vi "Update String Value.vi"(10 "Tree Tag":string, 11 "UI Data In":refnum<class "Settings UI.lvclass">) -> (2 "New Tree Value":string, 3 "UI Data Out":refnum<class "Settings UI.lvclass">)   [LabVIEW 2020, in "Output Sequencer.lvlib" / "Settings UI.lvclass"]
uses:
  Settings UI.lvclass
  Settings UI.lvclass/Settings UI.ctl
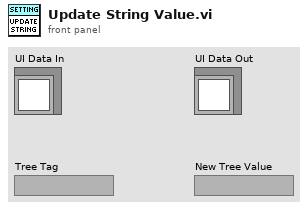
[diagram p1: front panel]
types:
  T1 = typedef "Output Sequencer.lvlib/Settings UI.lvclass/Tree Index Enum.ctl" = enum16{"General Settings", "Num Steps", "Num Analog", "Num Digital", "Show Confirmation", "Interp Priority", "Adv Timing", "Enable Conditions", "Seq Execution", "Reset Test Start", "Only When Test", "Delay After Test", "Start condition", "Re-triggering", "Stop condition", "Stop After Cycles", "Stop Values", "Default Values", "Default Analog", "Default Digital", "Steps", "Step #", "Description", "Precondition", "Duration", "Mode", "Delay Between Vals", "Analog Values", "Digital Values", "Postcondition", "On True", "On False"}
  T2 = typedef "Output Sequencer.lvlib/Settings UI.lvclass/Step Settings.ctl" = cluster{"Description":string, "Precondition":string, "Duration":dbl, "Mode":string, "Delay Between Values":dbl, "Analog Values":string[], "Digital Values":string[], "Postcondition":string, "On True":string, "On False":string}
  T3 = map{i32, cluster{"Step Number":i32, "Description":string}}
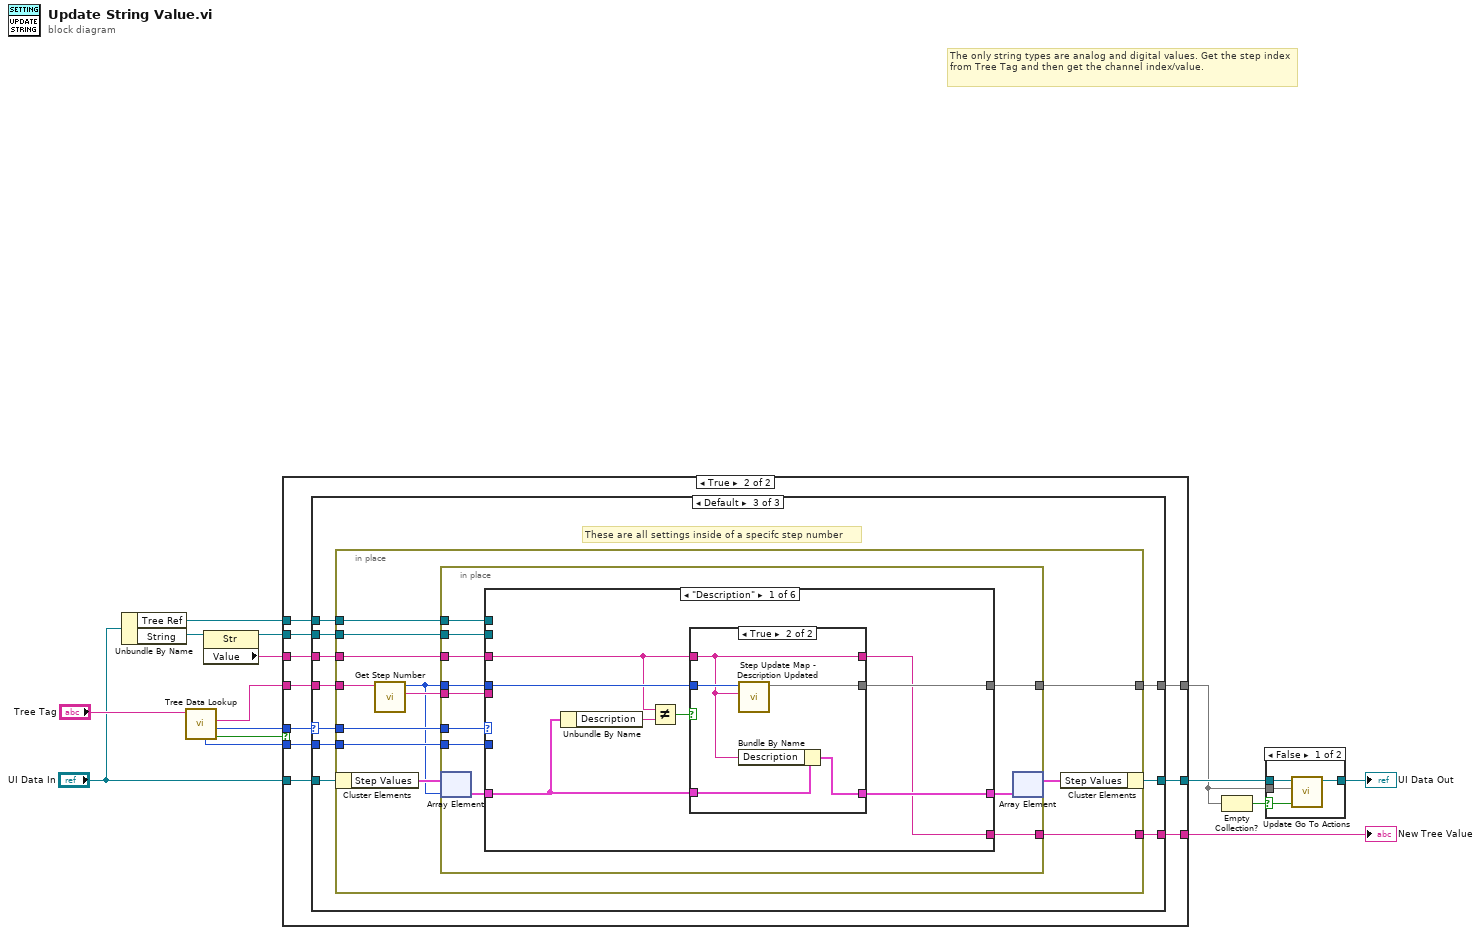
[diagram p0: block diagram]
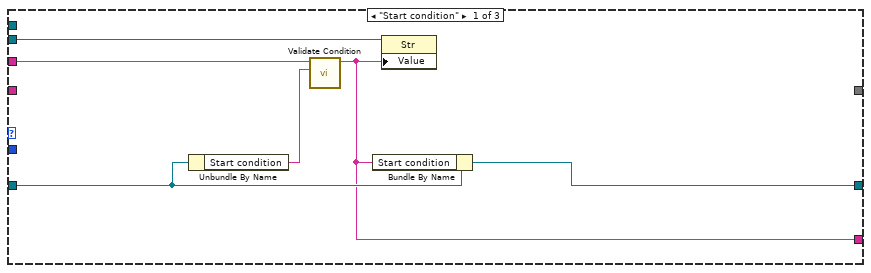
[diagram p4: hidden frame]
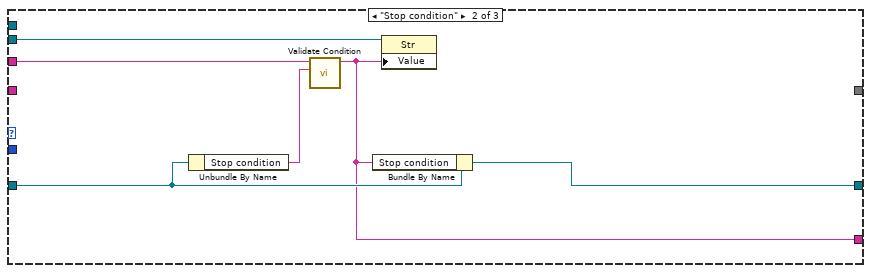
[diagram p5: hidden frame]
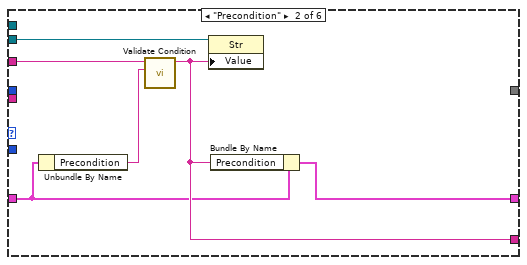
[diagram p7: hidden frame]
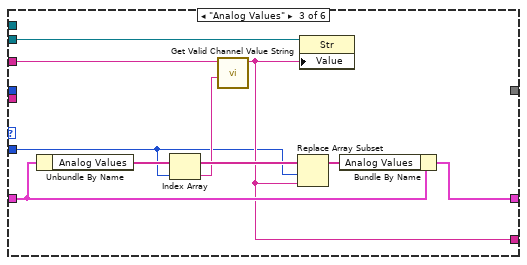
[diagram p8: hidden frame]
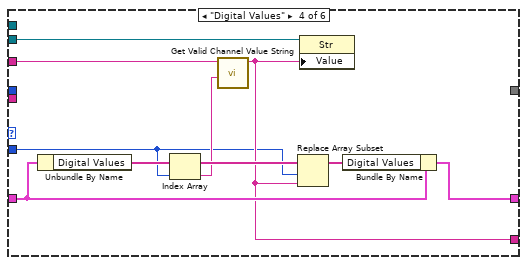
[diagram p9: hidden frame]
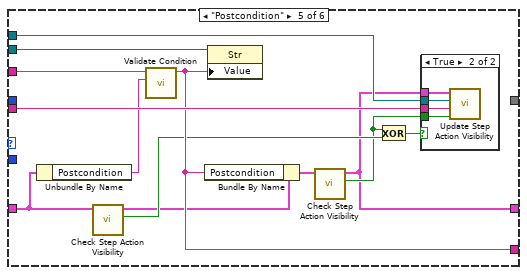
[diagram p10: hidden frame]
diagram:
  # "The only string types are analog and digital values. Get the step index from Tree Tag and then get the channel index/value."
  n1 = Unbundle By Name("UI Data In") -> ("Tree Ref"=w10:refnum<vi>, "String"=w13:refnum<vi>)
  n2 = call "Tree Data Lookup.vi"("Tag in"="Tree Tag") -> ("Found?"=w8:bool, "Tree Index Enum"=w9:T1, "Tag out"=w6:string, "Item Number"=w7:i32)  [unwired: 5 in, 2 out]
  n3 = property class="Str"(reference=w13) -> (reference out=w12:refnum<vi>, "Value"=w11:string)  [unwired: 1 in, 1 out]
  n4 = case shown="True" w8 {
    tunnel: "UI Data In" -> [w17 w27]
    tunnel: [w17 w26] -> w4
    tunnel: [w16 w25] -> w15
    tunnel: w12 -> [_ w24]
    tunnel: w11 -> [w16 w23]
    tunnel: w10 -> [_ w22]
    tunnel: w6 -> [_ w21]
    tunnel: w9 -> [_ w20]
    tunnel: w7 -> [_ w19]
    tunnel: [_ w18] -> w1
    frame False {
    }
    frame True {
      n5 = case shown="Default" w20 {
        selector: w20 -> [_ _ w44]
        tunnel: w27 -> [w31 w37 w42]
        tunnel: [w29 w35 w41] -> w26
        tunnel: [w30 w36 w49] -> w25
        tunnel: w24 -> [w28 w34 w48]
        tunnel: w23 -> [w32 w38 w47]
        tunnel: w22 -> [_ _ w46]
        tunnel: w21 -> [_ _ w45]
        tunnel: w19 -> [_ _ w43]
        tunnel: [_ _ w40] -> w18
        frame "Start condition" {
          n6 = Unbundle By Name(w31) -> ("Start condition"=w33:string)
          n7 = call "Validate Condition.vi"("Previous Condition"=w33, "Condition in"=w32) -> ("Valid Condition out"=w30:string)  [unwired: 9 in]
          n8 = Bundle By Name(cluster=w31, "Start condition"=w30) -> (w29:refnum<class "Settings UI.lvclass">)
          n9 = property class="Str"(reference=w28, "Value"=w30) -> ()  [unwired: 1 in, 2 out]
        }
        frame "Stop condition" {
          n10 = Unbundle By Name(w37) -> ("Stop condition"=w39:string)
          n11 = call "Validate Condition.vi"("Previous Condition"=w39, "Condition in"=w38) -> ("Valid Condition out"=w36:string)  [unwired: 9 in]
          n12 = Bundle By Name(cluster=w37, "Stop condition"=w36) -> (w35:refnum<class "Settings UI.lvclass">)
          n13 = property class="Str"(reference=w34, "Value"=w36) -> ()  [unwired: 1 in, 2 out]
        }
        frame Default {
          # "These are all settings inside of a specifc step number"
          n14 = in-place {
            in-place-border: [w61] -> w49
            in-place-border: w48 -> [w60]
            in-place-border: w47 -> [w59]
            in-place-border: w46 -> [w58]
            in-place-border: w45 -> [w57]
            in-place-border: w44 -> [w56]
            in-place-border: w43 -> [w55]
            in-place-border: [w51] -> w40
            n15 = in-place-cluster #1(w42) -> ("Step Values"=w53:T2[])
            n16 = call "Get Step Number.vi"("Tree Tag"=w57) -> ("Step tag"=w54:string, "Step Number"=w50:i32)  [unwired: 8 in, 1 out]
            n17 = in-place {
              in-place-border: w60 -> [w72]
              in-place-border: w59 -> [w71]
              in-place-border: [w70] -> w61
              in-place-border: w58 -> [w67]
              in-place-border: w54 -> [w66]
              in-place-border: w56 -> [w65]
              in-place-border: w55 -> [w64]
              in-place-border: [w63] -> w51
              in-place-border: w50 -> [w62]
              n18 = in-place-array #2(w53, w50) -> (w69:T2)
              n19 = case shown="\"Description\"" w65 {
                tunnel: w72 -> [_ w91 w100 w109 w121 _]
                tunnel: w71 -> [w75 w92 w99 w108 w122 w129]
                tunnel: [w73 w90 w96 w105 w120 w129] -> w70
                tunnel: w69 -> [w77 w89 w97 w106 w114 w130]
                tunnel: [w80 w93 w98 w107 w115 w130] -> w68
                tunnel: w67 -> [_ _ _ _ w124 _]
                tunnel: w66 -> [_ _ _ _ w123 _]
                tunnel: w64 -> [_ _ w94 w103 _ _]
                tunnel: [w79 _ _ _ _ _] -> w63
                tunnel: w62 -> [w78 _ _ _ _ _]
                frame "Description" {
                  n20 = Unbundle By Name(w77) -> ("Description"=w76:string)
                  n21 = Not Equal?(x=w75, y=w76) -> (x != y?=w74:bool)
                  n22 = case shown="True" w74 {
                    tunnel: [w81 w87] -> w80
                    tunnel: [_ w86] -> w79
                    tunnel: w78 -> [_ w85]
                    tunnel: w77 -> [w81 w84]
                    tunnel: w75 -> [w82 w83]
                    tunnel: [w82 w83] -> w73
                    frame False {
                    }
                    frame True {
                      n23 = call "Step Update Map - Description Updated.vi"("New Description"=w83, "Step Number"=w85) -> ("Step Update Map out"=w86:T3)  [unwired: 9 in]
                      n24 = Bundle By Name(cluster=w84, "Description"=w83) -> (w87:T2)
                    }
                  }
                }
                frame "Precondition" {
                  n25 = Unbundle By Name(w89) -> ("Precondition"=w88:string)
                  n26 = call "Validate Condition.vi"("Previous Condition"=w88, "Condition in"=w92) -> ("Valid Condition out"=w90:string)  [unwired: 9 in]
                  n27 = property class="Str"(reference=w91, "Value"=w90) -> ()  [unwired: 1 in, 2 out]
                  n28 = Bundle By Name(cluster=w89, "Precondition"=w90) -> (w93:T2)
                }
                frame "Analog Values" {
                  n29 = Unbundle By Name(w97) -> ("Analog Values"=w102:string[])
                  n30 = Index Array(array=w102, index=w94) -> (element=w101:string)
                  n31 = call "Get Valid Channel Value String.vi"("Previous Values"=w101, "Channel Values"=w99) -> ("Valid Channel Values"=w96:string)  [unwired: 9 in]
                  n32 = Replace Array Subset(array=w102, new element=w96, index=w94) -> (w95:string[])
                  n33 = property class="Str"(reference=w100, "Value"=w96) -> ()  [unwired: 1 in, 2 out]
                  n34 = Bundle By Name(cluster=w97, "Analog Values"=w95) -> (w98:T2)
                }
                frame "Digital Values" {
                  n35 = Unbundle By Name(w106) -> ("Digital Values"=w111:string[])
                  n36 = Index Array(array=w111, index=w103) -> (element=w110:string)
                  n37 = call "Get Valid Channel Value String.vi"("Previous Values"=w110, "Channel Values"=w108) -> ("Valid Channel Values"=w105:string)  [unwired: 9 in]
                  n38 = Replace Array Subset(array=w111, new element=w105, index=w103) -> (w104:string[])
                  n39 = property class="Str"(reference=w109, "Value"=w105) -> ()  [unwired: 1 in, 2 out]
                  n40 = Bundle By Name(cluster=w106, "Digital Values"=w104) -> (w107:T2)
                }
                frame "Postcondition" {
                  n41 = Unbundle By Name(w114) -> ("Postcondition"=w119:string)
                  n42 = call "Check Step Action Visibility.vi"("Step Settings in"=w114) -> ("Actions visible"=w118:bool, "Step Settings out"=w113:T2)  [unwired: 9 in]
                  n43 = call "Validate Condition.vi"("Previous Condition"=w119, "Condition in"=w122) -> ("Valid Condition out"=w120:string)  [unwired: 9 in]
                  n44 = Bundle By Name(cluster=w113, "Postcondition"=w120) -> (w112:T2)
                  n45 = property class="Str"(reference=w121, "Value"=w120) -> ()  [unwired: 1 in, 2 out]
                  n46 = call "Check Step Action Visibility.vi"("Step Settings in"=w112) -> ("Actions visible"=w116:bool, "Step Settings out"=w115:T2)  [unwired: 9 in]
                  n47 = Exclusive Or(1:w118, 2:w116) -> (0:w117:bool)
                  n48 = case shown="True" w117 {
                    tunnel: w124 -> [_ w127]
                    tunnel: w123 -> [_ w126]
                    tunnel: w115 -> [_ w128]
                    tunnel: w116 -> [_ w125]
                    frame False {
                    }
                    frame True {
                      n49 = call "Update Step Action Visibility.vi"("Actions visible"=w125, "Step tag"=w126, "TreeControl in"=w127, "Step Settings"=w128) -> ()  [unwired: 8 in]
                    }
                  }
                }
                frame Default {
                }
              }
              n50 = in-place-array #2(w68) -> (w52:T2[])  [unwired: 1 out]
            }
            n51 = in-place-cluster #1("Step Values"=w52) -> (w41:refnum<class "Settings UI.lvclass">)
          }
        }
      }
    }
  }
  "New Tree Value" <- w15
  n52 = Empty Collection?(1:w1) -> (0:w2:bool)
  n53 = case shown="False" w2 {
    selector: w2 -> [w131 _]
    tunnel: w4 -> [w134 w135]
    tunnel: [w133 w135] -> w3
    tunnel: w1 -> [w132 _]
    frame False {
      n54 = call "Update Go To Actions.vi"("Show Dialogs (default: True)"=w131, "Step Update Map in"=w132, "Settings UI in"=w134) -> ("Settings UI out"=w133:refnum<class "Settings UI.lvclass">)  [unwired: 8 in]
    }
    frame True {
    }
  }
  "UI Data Out" <- w3
